vi "Pockels Cal-Cal core.vi"(11 "Pockels power (%)":dbl(slide)=50.0 min=0.0 max=100.0 step=0.1 scale=0.0..100.0) -> (1 "Back-aperture power (mW)":dbl format="%#_gmW", 2 "Power after the objective (mW)":dbl, 3 "Pockels Volts":dbl format="%#_6fV")   [LabVIEW 2020]
uses:
  Typedefs/Functional global standard states.ctl
  Global Variables/gl_UI Ctrl Refs.vi
  <vilib>/gmath/NI_Gmath.lvlib
panel:
  out "Power (mW)":dbl[](array[numeric])
  out "Pockels V":dbl[](array[numeric])
  # "mW power at requested %"
  # "Pockels voltage for requested power."
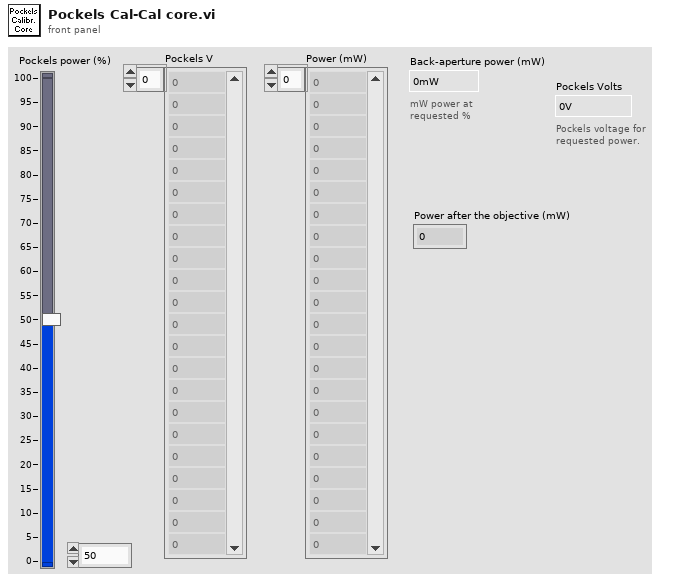
[diagram p1: front panel]
types:
  T1 = typedef "Functional global standard states.ctl" = enum16{"Initialise", "Read", "Write", "Load", "Save", "Clear"}
  T2 = cluster{"Start point index":i32, "End point index":i32}
  T3 = typedef "UI ctrl refs cluster.ctl" = cluster{"Top level VI path":path, "Top level VI ref":refnum<vi>, "User menu ref":refnum<k9>, "Sub Panel control":refnum<vi>, "Imaging Param Tab":refnum<vi>, "Occurrence-Start drivers":refnum<k4>, "Occurrence-Speed logging initialised":refnum<k4>, "Occurrence-XYZ stage initialised":refnum<k4>, "Exit button":refnum<vi>, "Status ind":refnum<vi>, "Set as origin":refnum<vi>, "Speed Logging":refnum<vi>, "Time Lapse":refnum<vi>, "Live Imaging":refnum<vi>, "AOL Z Stack":refnum<vi>, "Motor Z Stack":refnum<vi>, "Funct Acq button":refnum<vi>, "Hard Shutter":refnum<vi>, "Virtual Shutter":refnum<vi>, "Laser Power":refnum<vi>, "AOL Mode":refnum<vi>, "Frame Size":refnum<vi>, "Field of View":refnum<vi>, "Dwell Time":refnum<vi>, "Zoom":refnum<vi>, "AOL Z":refnum<vi>, "Objective":refnum<vi>, "Axis":refnum<vi>, "Paths & Names":refnum<vi>, "Experiment folder path (ind.)":refnum<vi>, "Last State (Ind.)":refnum<vi>, "Averages":refnum<vi>, "Angle (degrees)":refnum<vi>, "X centre":refnum<vi>, "Y centre":refnum<vi>, "Plane Mode":refnum<vi>, "# Planes":refnum<vi>, "Z Start":refnum<vi>, "Z Stop":refnum<vi>, "Z Step":refnum<vi>, "PMT 1":refnum<vi>, "PMT 2":refnum<vi>, "Stage XYZ Position":refnum<vi>, "Pockels@Z Start":refnum<vi>, "Pockels@Z Stop":refnum<vi>, "Obtain Z Start":refnum<vi>, "Obtain Z Stop":refnum<vi>, "Live stim.trig.period":refnum<vi>, "Live stim.trig.enable":refnum<vi>, "Movement Correction":refnum<vi>, "Load Reference Image":refnum<vi>, "XY Stage Move":refnum<vi>, "MovCor Cluster":refnum<vi>, "RefDAQParam":refnum<vi>, "Funct. Acq. Pockels Modulation":refnum<vi>, "Ref Laser Power":refnum<vi>, "Enable Video Recording":refnum<vi>, "Video Record-Live Imaging":refnum<vi>, "Video Record-Funct acq":refnum<vi>, "Reference Source":refnum<vi>, "AOL Z-stack Chirps Ready (ind)":refnum<vi>, "Target time between mov.cor. ref triggers (ms)":refnum<vi>, "Funct. Acq. Ref frame save":refnum<vi>, "Tracking button":refnum<vi>, "Show ref plots window":refnum<vi>, "Center freq ind (nm)":refnum<vi>, "Pickup mode (ind)":refnum<vi>, "Logging queue (ind)":refnum<vi>, "Back aperture power (ind.)":refnum<vi>, "Power after objective (ind.)":refnum<vi>, "Switch user":refnum<vi>, "Ls1 Conn. Status":refnum<vi>, "Ls1Tuning Status":refnum<vi>, "Ls1 Faults":refnum<vi>, "Ls1 Connection":refnum<vi>, "Ls1 Mode":refnum<vi>, "Ls1 POWER [mW]":refnum<vi>, "Ls1Shutter":refnum<vi>, "Ls1 Wavelength":refnum<vi>, "Ls1 Note":refnum<vi>, "Ls1 Confirm Wav":refnum<vi>, "Ls1 PreChrp Prism1":refnum<vi>, "Ls1 PreChrp Prism2":refnum<vi>, "Ls1 wav top Ind":refnum<vi>, "Ls1 power top Ind":refnum<vi>, "Ls1 Pump peak Hold":refnum<vi>, "Ls1 Status Ind":refnum<vi>, "Ls1 wav cancel":refnum<vi>, "Experiment Type":refnum<vi>, "Biology Information":refnum<vi>, "Camera recording status":refnum<vi>}
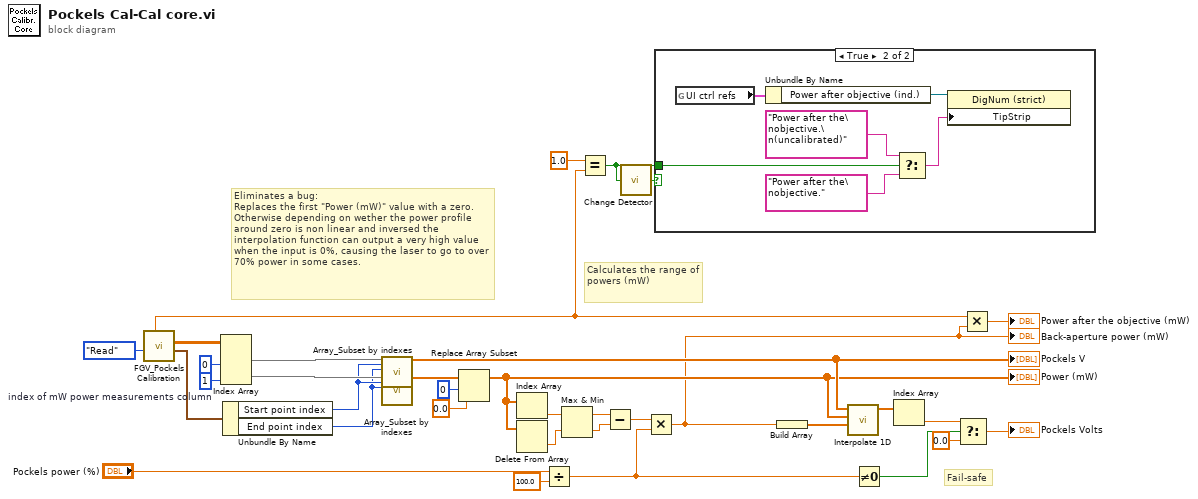
[diagram p0: block diagram]
diagram:
  w22 = 1  # index of mW power measurements column
  # "Fail-safe"
  # "Eliminates a bug:\nReplaces the first \"Power (mW)\" value with a zero. Otherwise depending on wether the power profile around zero is non linear and inversed the interpolation function can output a very high value when the input is 0%, causing the laser to go to over 70% power in some cases."
  # "Calculates the range of powers (mW)"
  n1 = call "FGV_Pockels Calibration.vi"("Function"=Functional_global_standard_states."Read") -> ("Cal subset indexes"=w18:T2, "Pockels calibration data (Single wavelength)"=w31:dbl[][], "Multiplier for power after the objective"=w4:dbl)  [unwired: 4 in, 4 out]
  n2 = Index Array(array=w31, index (col) #1=0 ("disabled index (col)"), index (col) #2=w22) -> (element #1=w20:dbl[], element #2=w21:dbl[])  [unwired: 2 in]
  n3 = Unbundle By Name(w18) -> ("Start point index"=w17:i32, "End point index"=w16:i32)
  n4 = call "Array_Subset by indexes.vi"("Array in"=w20, "Start point index"=w17, "End point index"=w16) -> ("Array out"=w19:dbl[])  [unwired: 16 in]
  "Pockels V" <- w19
  n5 = call "Array_Subset by indexes.vi"("Array in"=w21, "Start point index"=w17, "End point index"=w16) -> ("Array out"=w14:dbl[])  [unwired: 16 in]
  n6 = Replace Array Subset(array=w14, new element=0.0 ("new element/subarray"), index=0) -> (w13:dbl[])
  "Power (mW)" <- w13
  n7 = Index Array(array=w13) -> (element=w30:dbl)  [unwired: 1 in]
  n8 = Delete From Array(array=w13) -> (deleted portion=w29:dbl)  [unwired: 2 in, 1 out]
  n9 = Divide(x="Pockels power (%)", y=100.0) -> (x/y=w11:dbl)
  n10 = Max & Min(x=w30, y=w29) -> (max(x,y)=w28:dbl, min(x,y)=w27:dbl)
  n11 = Equal?(x=1.0, y=w4) -> (x = y?=w1:bool)
  n12 = Subtract(x=w28, y=w27) -> (x-y=w24:dbl)
  n13 = call <userlib>:"Change Detector.vi"("Value"=w1) -> ("Changed?"=w2:bool)
  n14 = Multiply(x=w24, y=w11) -> (x*y=w5:dbl)
  "Back-aperture power (mW)" <- w5
  n15 = case shown="True" w2 {
    tunnel: w1 -> [_ w36]
    frame False {
    }
    frame True {
      n16 = global read "gl_UI Ctrl Refs.vi" "UI ctrl refs"() -> (w39:T3)
      n17 = Unbundle By Name(w39) -> ("Power after objective (ind.)"=w40:refnum<vi>)
      n18 = Select(t="Power after the\nobjective.\n(uncalibrated)" ("Tip Strip"), s=w36, f="Power after the\nobjective." ("Tip Strip")) -> (s? t:f=w37:string)
      n19 = property class="DigNum (strict)"(reference=w40, "TipStrip"=w37) -> ()  [unwired: 1 in, 2 out]
    }
  }
  n20 = Build Array(w5) -> (w33:dbl[])
  n21 = call <vilib>:"Interpolate 1D.vi"("xi"=w33, "X"=w13, "Y"=w19) -> ("yi"=w34:dbl[])  [unwired: 6 in, 2 out]
  n22 = Not Equal To 0?(x=w11) -> (x != 0?=w8:bool)
  n23 = Index Array(array=w34) -> (element=w10:dbl)  [unwired: 1 in]
  n24 = Select(t=w10, s=w8, f=0.0) -> (s? t:f=→"Pockels Volts":dbl)
  n25 = Multiply(x=w4, y=w5) -> (x*y=→"Power after the objective (mW)":dbl)
